vi "Simple SCP File Upload.vi"() -> ()   [LabVIEW 2018]
doc: "Uploads, or sends, a relatively small local file to a remote SSH server. This is similar to the SCP command line utility when transferring, or copying, a local file to a remote destination. If performance is poor or memory is limited on the local machine, then it could be because the file is relatively large and this implementation is not very efficient for relatively large files."
uses:
  Toolkit/Type Definitions/Permissions.ctl
  Toolkit/Type Definitions/Modes.ctl
  Toolkit/Session/Support/Password Authentication.vi
  Toolkit/Channel/Support/Create from SCP Send.vi
  Toolkit/Channel/Support/Destroy to Session.vi
  Toolkit/SSH/SSH.lvclass
  Toolkit/Session/Session.lvclass
  Toolkit/Channel/Channel.lvclass
  Toolkit/Toolkit.lvlib
panel:
  in  "Remote File":string
  in  "Local File":path
  in  "Remote SSH Server":string
  in  "Password":string
  in  "Username":string
  # "Overview: Demonstrates transferring, or uploading, a local file to a remote SSH server, similar to the SCP command line utility\nInstructions:\n1. Enter the IP address or host name of the remote SSH server. This can be a CompactRIO (cRIO) running the National Instruments Linux Real-Time (NI Linux RT) operating system with the Enable Secure Shell Server (sshd) checkbox checked. \n2. Enter a username. If using a cRIO with a default configuration, then the username is \"admin\".\n3. Enter a password for the username. If using a cRIO with a default configuration, then the password is blank (empty).\n4. Select a file on the local computer to transfer/upload to the remote SSH server.\n5. Enter a path and/or filename for the uploaded file on the remote SSH server. Typically, this is a POSIX/UNIX file path with a backslash, \"/\", use to separate directories and the default directory is the remote user's home directory, i.e. \"/home/admin\" on a default configured cRIO.\n6. Run this VI."
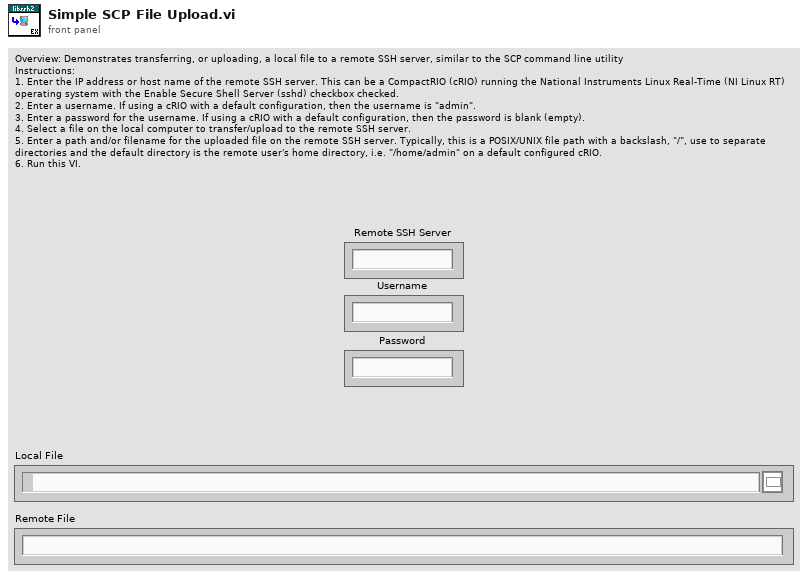
[diagram p1: front panel]
types:
  T1 = enum16{"open", "replace", "create", "open or create", "replace or create", "replace or create with confirmation"}
  T2 = typedef "Toolkit.lvlib/Permissions.ctl" = cluster{"Owner":T3, "Group":T3, "Others":T3}
  T3 = typedef "Toolkit.lvlib/Modes.ctl" = cluster{"Read":bool, "Write":bool, "Execute":bool}
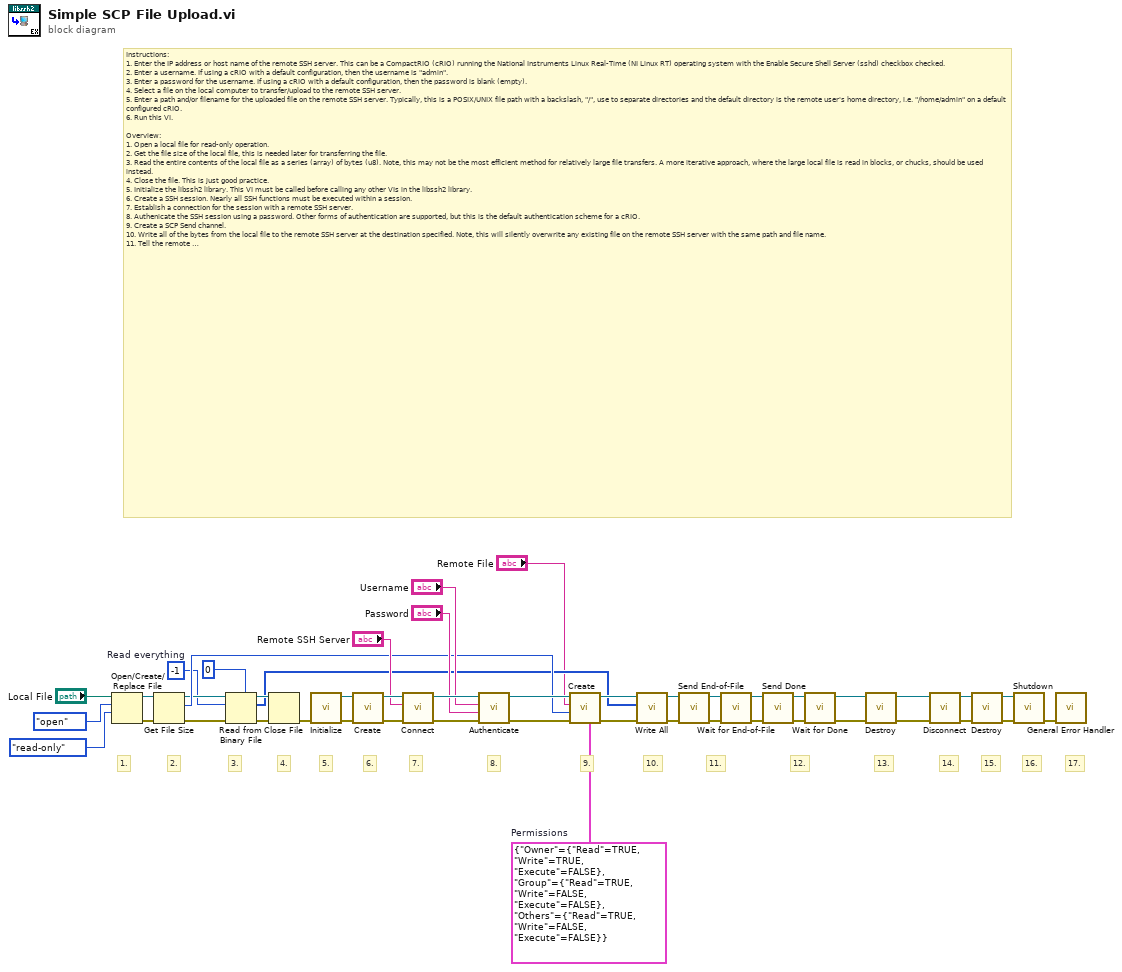
[diagram p0: block diagram]
diagram:
  w30 = -1  # Read everything
  w32 = T2 {"Owner"={"Read"=TRUE, "Write"=TRUE, "Execute"=FALSE}, "Group"={"Read"=TRUE, "Write"=FALSE, "Execute"=FALSE}, "Others"={"Read"=TRUE, "Write"=FALSE, "Execute"=FALSE}}  # Permissions
  # "17."
  # "16."
  # "15."
  # "14."
  # "13."
  # "12."
  # "11."
  # "10."
  # "9."
  # "8."
  # "7."
  # "6."
  # "5."
  # "4."
  # "3."
  # "2."
  # "1."
  # "Instructions:\n1. Enter the IP address or host name of the remote SSH server. This can be a CompactRIO (cRIO) running the National Instruments Linux Real-Time (NI Linux RT) operating system with the Enable Secure Shell Server (sshd) checkbox checked. \n2. Enter a username. If using a cRIO with a default configuration, then the username is \"admin\".\n3. Enter a password for the username. If using a cRIO with a default configuration, then the password is blank (empty).\n4. Select a file on the local computer to transfer/upload to the remote SSH server.\n5. Enter a path and/or filename for the uploaded file on the remote SSH server. Typically, this is a POSIX/UNIX file path with a backslash, \"/\", use to separate directories and the default directory is the remote user's home directory, i.e. \"/home/admin\" on a default configured cRIO.\n6. Run this VI.\n\nOverview:\n1. Open a local file for read-only operation.\n2. Get the file size of the local file, this is needed later for transferring the file.\n3. Read the entire contents of the local file as a series (array) of bytes (u8). Note, this may not be the most efficient method for relatively large file transfers. A more iterative approach, where the large local file is read in blocks, or chucks, should be used instead.\n4. Close the file. This is just good practice.\n5. Initialize the libssh2 library. This VI must be called before calling any other VIs in the libssh2 library.\n6. Create a SSH session. Nearly all SSH functions must be executed within a session.\n7. Establish a connection for the session with a remote SSH server.\n8. Authenicate the SSH session using a password. Other forms of authentication are supported, but this is the default authentication scheme for a cRIO. \n9. Create a SCP Send channel.\n10. Write all of the bytes from the local file to the remote SSH server at the destination specified. Note, this will silently overwrite any existing file on the remote SSH server with the same path and file name.\n11. Tell the remote SSH server that all of the bytes from the local file have been sent to it and no more bytes will be sent. Also, wait for the remote SSH server to acknowledge that the file transfer is complete. This is not strictly required, but it is good practice.\n12. Signal completion of the SCP Send channel to the remote server. Again, not strictly required, but it is good practice.\n13. Destroy the SCP Send channel. Since the \"Create\" VI is used, the complementary \"Destroy\" VI must be used to free resources within the libssh2 library.\n14. Disconnect from the remote SSH server.\n15. Destroy the session to free resources within the libssh2 library.\n16. Shutdown the libssh2 library. This VI must be last VI called for the libssh2 library. No other libssh2 VIs should be called once this VI is executed.\n17. Provide some error handling and reporting. Libssh2 errors will be in the -8100 range."
  n1 = Open/Create/Replace File(file path (use dialog)="Local File", operation (0:open)=T1."open", access (0:read/write)=enum16{"read/write", "read-only", "write-only"}."read-only") -> (refnum out=w34:refnum<file>, error out=w35:errorcluster)  [unwired: 3 in, 1 out]
  n2 = Get File Size(file=w34, error in=w35) -> (refnum out=w31:refnum<file>, size (in bytes)=w33:i64, 0:w28:errorcluster)
  n3 = Read from Binary File(5:u8 0, 8:w28, 10:w30, 11:w31) -> (0:w26:errorcluster, 2:w5:u8[], 3:w27:refnum<file>)  [unwired: 2 in, 1 out]
  n4 = Close File(refnum=w27, error in=w26) -> (error out=w25:errorcluster)  [unwired: 1 out]
  n5 = call "Initialize.vi"("Error In"=w25) -> ("Error Out"=w45:errorcluster, "SSH"=w46:refnum<class "SSH.lvclass">)  [unwired: 9 in]
  n6 = call "Create.vi"("Error In"=w45, "SSH"=w46) -> ("Error Out"=w43:errorcluster, "Sesssion"=w44:refnum<class "Session.lvclass">)  [unwired: 8 in]
  n7 = call "Connect.vi"("Error In"=w43, "Address"="Remote SSH Server", "Session In"=w44) -> ("Error Out"=w41:errorcluster, "Sesssion Out"=w42:refnum<class "Session.lvclass">)  [unwired: 7 in]
  n8 = call-poly "Authenticate.vi"("Error In"=w41, "Password"="Password", "Username"="Username", "Session In"=w42) -> ("Error Out"=w36:errorcluster, "Sesssion Out"=w37:refnum<class "Session.lvclass">)  [unwired: 6 in]
  n9 = call-poly "Create.vi"("Permissions"=w32, "Error In"=w36, "File Size"=w33, "Remote Destination Path"="Remote File", "Session"=w37) -> ("Error Out"=w8:errorcluster, "Channel"=w9:refnum<class "Channel.lvclass">)  [unwired: 5 in]
  n10 = call "Write All.vi"("Error In"=w8, "Data"=w5, "Channel In"=w9) -> ("Error Out"=w6:errorcluster, "Channel Out"=w7:refnum<class "Channel.lvclass">)  [unwired: 6 in, 1 out]
  n11 = call "Send End-of-File.vi"("Error In"=w6, "Channel In"=w7) -> ("Error Out"=w23:errorcluster, "Channel Out"=w24:refnum<class "Channel.lvclass">)  [unwired: 8 in]
  n12 = call "Wait for End-of-File.vi"("Error In"=w23, "Channel In"=w24) -> ("Error Out"=w14:errorcluster, "Channel Out"=w15:refnum<class "Channel.lvclass">)  [unwired: 8 in]
  n13 = call "Send Done.vi"("Error In"=w14, "Channel In"=w15) -> ("Error Out"=w12:errorcluster, "Channel Out"=w13:refnum<class "Channel.lvclass">)  [unwired: 8 in]
  n14 = call "Wait for Done.vi"("Error In"=w12, "Channel In"=w13) -> ("Error Out"=w10:errorcluster, "Channel Out"=w11:refnum<class "Channel.lvclass">)  [unwired: 8 in]
  n15 = call-poly "Destroy.vi"("Error In"=w10, "Channel"=w11) -> ("Error Out"=w21:errorcluster, "Session"=w22:refnum<class "Session.lvclass">)  [unwired: 8 in]
  n16 = call "Disconnect.vi"("Error In"=w21, "Session In"=w22) -> ("Error Out"=w19:errorcluster, "Sesssion Out"=w20:refnum<class "Session.lvclass">)  [unwired: 8 in]
  n17 = call "Destroy.vi"("Error In"=w19, "Session"=w20) -> ("Error Out"=w17:errorcluster, "SSH"=w18:refnum<class "SSH.lvclass">)  [unwired: 8 in]
  n18 = call "Shutdown.vi"("Error In"=w17, "SSH"=w18) -> ("Error Out"=w16:errorcluster)  [unwired: 9 in]
  n19 = call <vilib>:"General Error Handler.vi"("error in (no error)"=w16) -> ()  [unwired: 10 in, 5 out]
